vi "Auth Extra.vi"(8 "error in (no error)":errorcluster, 10 "authextra in":string="{}", 11 "WampScramAuthenticator in":refnum<class "WampScramAuthenticator.lvclass">) -> (0 "error out":errorcluster, 2 "authextra out":string="{}", 3 "WampScramAuthenticator out":refnum<class "WampScramAuthenticator.lvclass">)   [LabVIEW 2020, in "wamplv.lvlib" / "WampScramAuthenticator.lvclass"]
uses:
  WampScramAuthenticator.lvclass
  6983e17e-729a-446d-8f72-2963547dcf6e.vi
  <vilib>/JDP Science/JSONtext/Variant to JSON Text.vi
  <vilib>/JDP Science/JSONtext/LVClass Serializer/JSONtext LVClass Serializer.lvclass
  WampScramAuthenticator.lvclass/WampScramAuthenticator.ctl
  <vilib>/JDP Science/JSONtext/JSONtext.lvlib
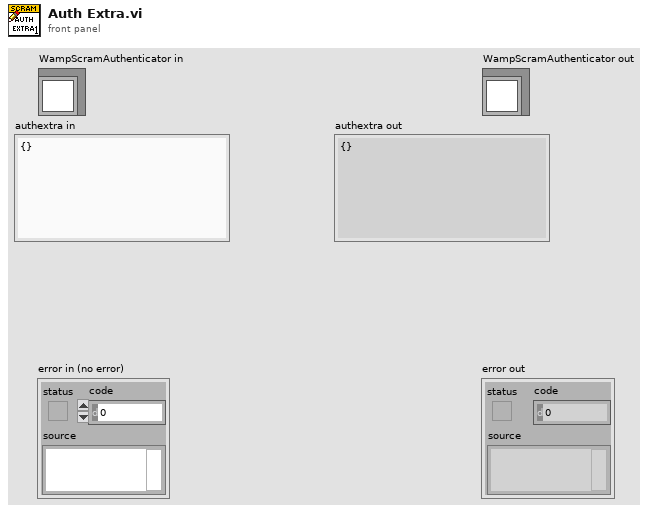
[diagram p1: front panel]
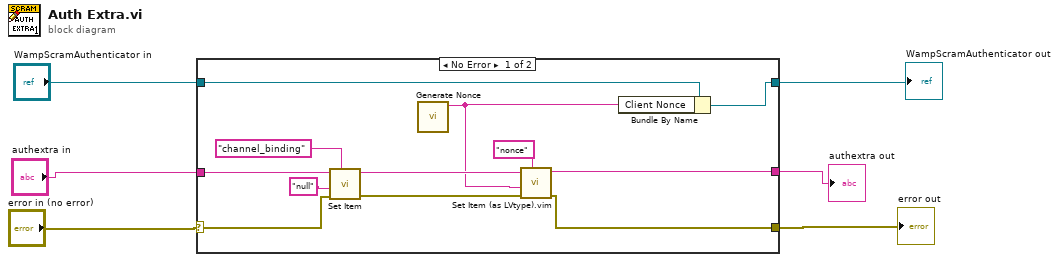
[diagram p0: block diagram]
diagram:
  n1 = case shown="No Error" "error in (no error)" {
    selector: "error in (no error)" -> [w15 w21]
    tunnel: [w13 w21] -> w5
    tunnel: "WampScramAuthenticator in" -> [w9 w20]
    tunnel: [w7 w20] -> w3
    tunnel: "authextra in" -> [w16 w19]
    tunnel: [w10 w19] -> w1
    frame No Error {
      n2 = call <vilib>:"Set Item.vi"("$Path or Item Name"="channel_binding", "error in (no error)"=w15, "JSON to Insert"="null", "JSON"=w16) -> ("error out"=w14:errorcluster, "<JSON>"=w11:string)  [unwired: 4 in, 1 out]
      n3 = call "Generate Nonce.vi"() -> ("Noce"=w8:string)  [unwired: 11 in]
      n4 = call "Set Item (as LVtype).vim"("$Path or Item Name"="nonce", "error in (no error)"=w14, "Anything"=w8, "JSON"=w11) -> ("error out"=w13:errorcluster, "<JSON>"=w10:string)  [unwired: 4 in, 1 out]
      n5 = Bundle By Name(cluster=w9, "Client Nonce"=w8) -> (w7:refnum<class "WampScramAuthenticator.lvclass">)
    }
    frame Error {
    }
  }
  "error out" <- w5
  "WampScramAuthenticator out" <- w3
  "authextra out" <- w1
